vi "Temperature Monitor.vi"() -> ()   [LabVIEW 2014]
doc: "This VI uses a While Loop and shift registers to average data. No hardware is necessary."
panel:
  in  "Stop Button":bool
  out "Temperature History":dbl(graph)
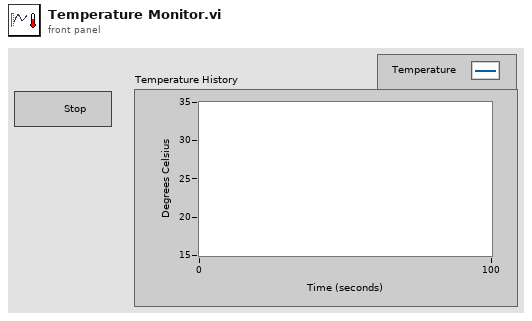
[diagram p1: front panel]
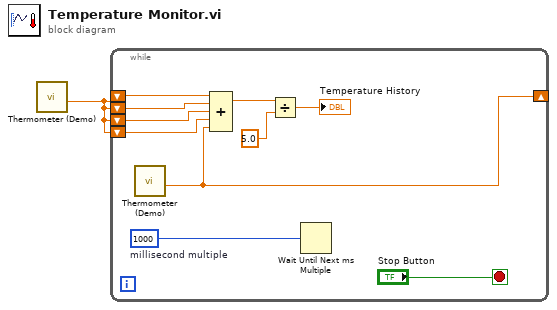
[diagram p0: block diagram]
diagram:
  n1 = call "Thermometer (Demo).vi"() -> ("Temperature Value"=w1:dbl)  [unwired: 11 in]
  n2 = while {
    shift-right: [w6] -> _
    shift-left: w1 -> [w10]
    shift-left: w1 -> [w9]
    shift-left: w1 -> [w5]
    shift-left: w1 -> [w4]
    stop <- "Stop Button" stop-if-true
    w11 = u32 1000  # millisecond multiple
    n3 = call "Thermometer (Demo).vi"() -> ("Temperature Value"=w6:dbl)  [unwired: 11 in]
    n4 = Compound Arithmetic op=ADD(w10, w9, w5, w4, w6) -> (w8:dbl)
    n5 = Divide(x=w8, y=5.0) -> (x/y=→"Temperature History":dbl)
    n6 = Wait Until Next ms Multiple(millisecond multiple=w11) -> ()  [unwired: 1 out]
  }
